vi "Clear Path.vi"(9 "Hallway in":string[](array[string]), 10 "Hallway Position in":i32, 11 "Room in":string) -> (0 "Clear Path?":bool, 1 "Hallway out":string[](array[string]), 2 "Hallway Position out":i32, 3 "Room out":string)   [LabVIEW 2019, in "23.lvlib" / "State.lvclass"]
uses:
  State.lvclass
  Destination Room Position.vi
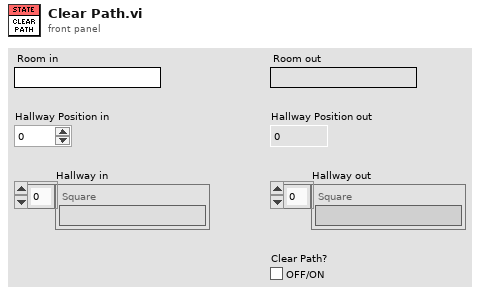
[diagram p1: front panel]
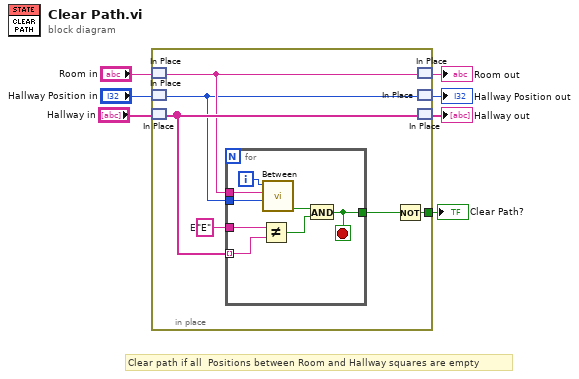
[diagram p0: block diagram]
diagram:
  # "Clear path if all  Positions between Room and Hallway squares are empty"
  n1 = in-place {
    in-place-border: [w13] -> w7
    w11 = "E"  # E
    n2 = in-place-match #1("Room in") -> (w9:string)
    n3 = in-place-match #2("Hallway Position in") -> (w8:i32)
    n4 = in-place-match #3("Hallway in") -> (w10:string[])
    n5 = for {
      tunnel: w10 -> [w14] mode=indexing
      tunnel: w8 -> [w20]
      tunnel: w9 -> [w19]
      tunnel: w11 -> [w18]
      tunnel: [w16] -> w12
      i -> [w21]
      stop <- w16 stop-if-true
      n6 = Not Equal?(x=w18, y=w14) -> (x != y?=w17:bool)
      n7 = call "Between.vi"("Hallway Position in"=w20, "Room in"=w19, "Position in"=w21) -> ("Betwwen?"=w15:bool)  [unwired: 5 in, 3 out]
      n8 = And(x=w15, y=w17) -> (x .and. y?=w16:bool)
    }
    n9 = Not(x=w12) -> (.not. x?=w13:bool)
    n10 = in-place-match #1(w9) -> (→"Room out":string)
    n11 = in-place-match #2(w8) -> (→"Hallway Position out":i32)
    n12 = in-place-match #3(w10) -> (→"Hallway out":string[])
  }
  "Clear Path?" <- w7
